vi "ProdaNG.Example.GetWabcoPartsOfProductionLine.vi"() -> ()   [LabVIEW 2016]
uses:
  Configurator/ProdaNG.Configurator.DB.ctl
panel:
  in  "DB":T1=enum."WPL"
  in  "Prod Line":string
  out "Wabco Parts":string[](array[string])
  in  "Connection string":string="lcptb/lcptb@proda_wpk"
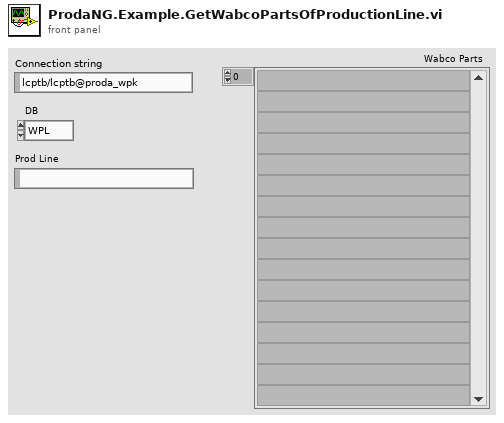
[diagram p1: front panel]
types:
  T1 = typedef "ProdaNG.Configurator.DB.ctl" = enum16{"other", "WPL", "WPK"}
  T2 = typedef "ProdaNG.WabcoPart.ctl" = cluster{"i_id":i32, "workCenterId":i32, "contentId":string, "previewId":string, "mdReason":string, "mdUser":string, "mdTime":string, "productName":string, "wabcoNumber":string}
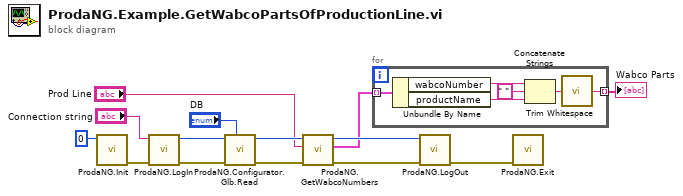
[diagram p0: block diagram]
diagram:
  n1 = call "ProdaNG.Init.vi"("numContexts (0: unlimited)"=0 ("numContexts")) -> ("error out"=w13:errorcluster)  [unwired: 10 in]
  n2 = call "ProdaNG.LogIn.vi"("error in"=w13, "ConnectionString"="Connection string") -> ("error out"=w3:errorcluster, "dbHandle"=w9:i32)  [unwired: 7 in, 1 out]
  n3 = call "ProdaNG.Configurator.Glb.Read.vi"("DB"="DB", "error in (no error)"=w3) -> ("error out"=w2:errorcluster)  [unwired: 7 in, 2 out]
  n4 = call "ProdaNG.GetWabcoNumbers.vi"("error in (no error)"=w2, "Production Line"="Prod Line", "dbHandle"=w9) -> ("error out"=w8:errorcluster, "WabcoParts"=w6:T2[], "dbHandle"=w7:i32)  [unwired: 5 in, 1 out]
  n5 = for {
    tunnel: w6 -> [w19] mode=indexing
    tunnel: [w14] -> w5 mode=indexing
    n6 = Unbundle By Name(w19) -> ("wabcoNumber"=w16:string, "productName"=w18:string)
    n7 = Concatenate Strings(w16, " " ("string"), w18) -> (w17:string)
    n8 = call <vilib>:"Trim Whitespace.vi"("string"=w17) -> ("trimmed string"=w14:string)  [unwired: 1 in]
  }
  "Wabco Parts" <- w5
  n9 = call "ProdaNG.LogOut.vi"("error in"=w8, "dbHandleIn"=w7) -> ("error out"=w11:errorcluster)  [unwired: 9 in]
  n10 = call "ProdaNG.Exit.vi"("error in (no error)"=w11) -> ()  [unwired: 10 in, 1 out]
